vi "Force Channel.vi"(7 "Plugin Name":string, 8 "error in (no error)":errorcluster, 9 "Force Channel":T1, 10 "Index":i32, 11 "CIF_Plugin_UI in":refnum<class "CIF_Plugin_UI.lvclass">) -> (0 "error out":errorcluster, 1 "Not Found":bool, 3 "CIF_Plugin_UI out":refnum<class "CIF_Plugin_UI.lvclass">)   [LabVIEW 2021, in "CIF_Plugin_UI.lvclass"]
uses:
  CIF_Plugin_UI.lvclass
  D:/dev/CIF-LVCore/src/CIFUI/CIF_UI.lvclass
  Typedef/Force Channel.ctl
  CIFCore/Grpc/CIFCoreChannel_client/RPC Messages/cif_channelcore_ForceChannel.ctl
  CIFUI/CIF_UI.lvclass
  CIFCore/Grpc/CIFCoreWrapper/CIFCoreWrapper.lvlib
  CIFCore/Grpc/CIFCoreChannel_client/CIFCoreChannel_client.lvlib
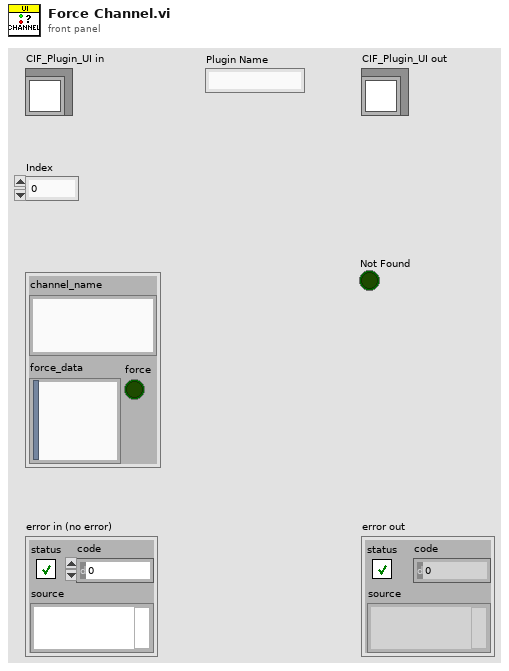
[diagram p1: front panel]
types:
  T1 = typedef "CIF_Plugin_UI.lvclass/Force Channel.ctl" = cluster{"channel_name":string, "force":bool, "force_data":string}
  T2 = typedef "CIFCoreChannel_client.lvlib/cif_channelcore_ForceChannel.ctl" = cluster{"channel_name":string, "force":bool, "force_data":u8[]}
  T3 = typedef "grpc-lvsupport-release.lvlib/grpcId.ctl" = u64
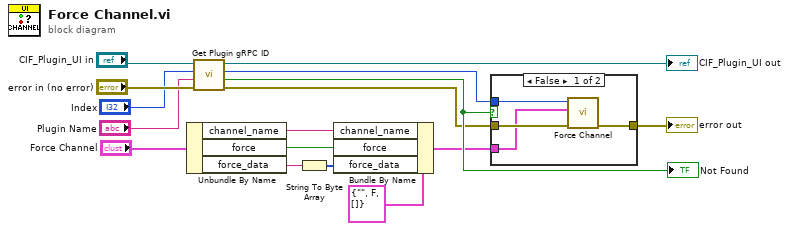
[diagram p0: block diagram]
diagram:
  n1 = Unbundle By Name("Force Channel") -> ("channel_name"=w3:string, "force"=w4:bool, "force_data"=w6:string)
  n2 = call "Get Plugin gRPC ID.vi"("error in (no error)"="error in (no error)", "Plugin Name"="Plugin Name", "Index"="Index", "CIF_UI in"="CIF_Plugin_UI in") -> ("error out"=w10:errorcluster, "Not Found"=w11:bool, "gRPC ID"=w12:T3, "CIF_UI out"=→"CIF_Plugin_UI out":refnum<class "CIF_Plugin_UI.lvclass">)  [unwired: 4 in]
  "Not Found" <- w11
  n3 = String To Byte Array(string=w6) -> (unsigned byte array=w5:u8[])
  n4 = Bundle By Name(cluster=T2 {"channel_name"="", "force"=FALSE, "force_data"=[]} ("Force Channel"), "channel_name"=w3, "force"=w4, "force_data"=w5) -> (w1:T2)
  n5 = case shown="False" w11 {
    tunnel: w12 -> [w20 _]
    tunnel: w10 -> [w19 w21]
    tunnel: [w18 w21] -> w9
    tunnel: w1 -> [w17 _]
    frame False {
      n6 = call "Force Channel.vi"("error in"=w19, "Force Channel"=w17, "gRPC ID"=w20) -> ("error out"=w18:errorcluster)  [unwired: 7 in, 1 out]
    }
    frame True {
    }
  }
  "error out" <- w9
